vi "prerequisites_to_start_sleep_detection.vi"(4 "Input \nparameters":T3={"Frame rate (ms)"=2000, "Worm strain"="N2", "Time t"=0, "State"=enum."Image acquisition", "Acquisition time"=0, "Max_num_runs"=100000, "#TTL"=0, "SD start reference time"=100000, "ImSub Value"=0, "Time of last TTL"=0, "Number of Columns"=2, "Number of Rows"=2, "# AdjacentTTL"=0, "Start sleep detection"="", "Sleep Detection"=FALSE, "# Sleep detections"=0, "Time of first sleep detection"=0, "Time max # adjacent TTL"=0, "Image t-1"=[], "Image t"=[]} {"Number of Rows" items=["1"=1, "2"=2, "3"=3, "4"=4]; "Number of Columns" items=["1"=1, "2"=2, "3"=3, "4"=4]}, 6 "Deprivation\nparameters":T1={"Frame Row"=0, "Kstd"=40.0, "# Images for\nsleep detection"=10, "Kmean"=1.5, "Start time of sleep detection"=1000, 0, "Max deprivation length"=3600, "Max # TTL"=10000, "Delay detection start by x images after first detection"=0, "Minimum Interval between TTL pulses"=0, "Delay sleep detection\nby x detections"=9, "# Total immobility\n detections"=0.0, "Pause max # adjacent\nTTL"=0, "TTL x start\ntime deprivation\n"=0.0, "Max #\nadjacent TTL"=10000, " Ca2+\nmode"=0} {"?" items=["1", "2", "3", "4"]; "Frame Row" items=["1", "2", "3", "4"]}) -> (1 "Output \nparameters":T4={"Frame rate (ms)"=2000, "Worm strain"="N2", "Time t"=0, "State"=enum."Image acquisition", "Time elapsed"=0.0, "Max_num_runs"=100000, "#TTL"=0, "SD start reference"=100000, "ImSub Value"=0, "Time of last TTL"=0, "Number of Columns"=2, "Number of Rows"=2, "# AdjacentTTL"=0, "Start sleep detection"="", "Sleep Detection"=FALSE, "# Sleep detections"=0, "Time of first sleep detection"=0, "Time max # adjacent TTL"=0, "Image t-1"=[], "Image t"=[]} {"Number of Rows" items=["1"=1, "2"=2, "3"=3, "4"=4]; "Number of Columns" items=["1"=1, "2"=2, "3"=3, "4"=4]})   [LabVIEW 2011]
uses:
  state.ctl
panel:
  # "Sleep deprivation settings"
  # "Select deprivation animal"
  # "Deprive image in row"
  # "Deprive image in column"
  # "Sleep detection parameters"
  # "Sleep deprivation parameters"
  # "Delay deprivation start:"
  # "Pause deprivation (images):"
  # "Stop deprivation after:"
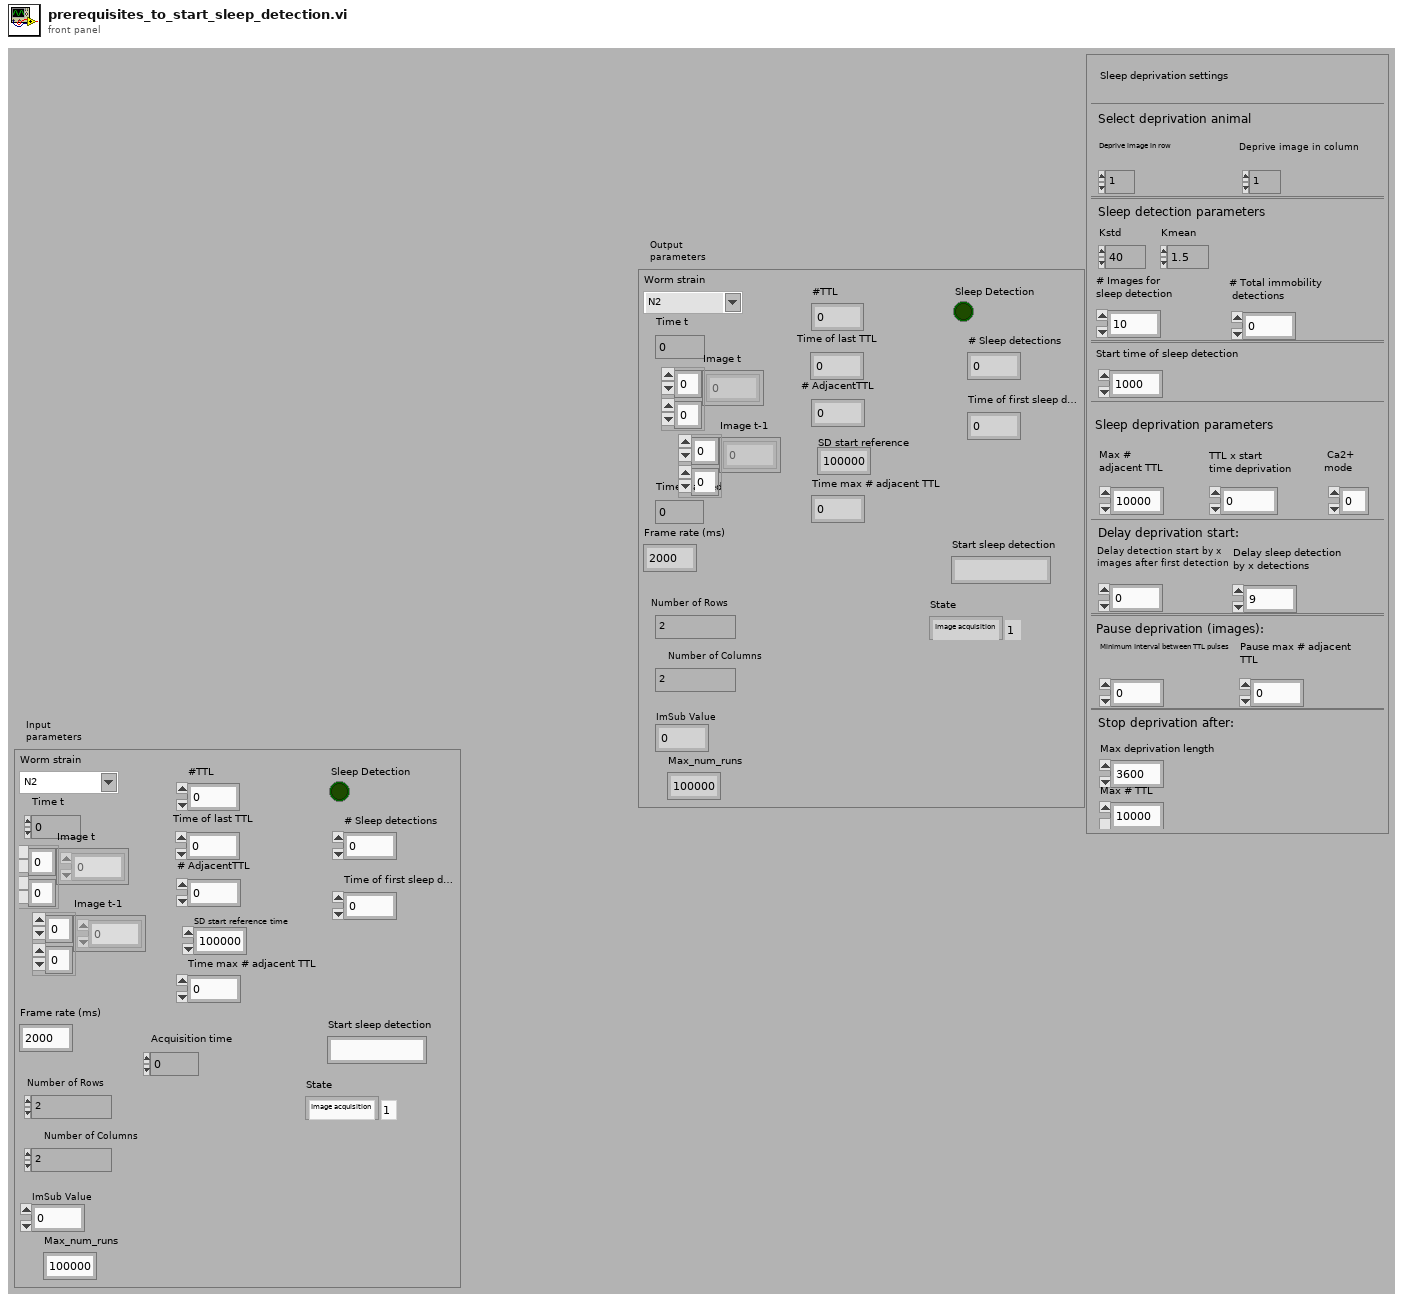
[diagram p1: front panel]
types:
  T1 = cluster{"Frame Row":u32, "Kstd":dbl, "# Images for\nsleep detection":i32, "Kmean":dbl, "Start time of sleep detection":i32, u32, "Max deprivation length":i32, "Max # TTL":i32, "Delay detection start by x images after first detection":i32, "Minimum Interval between TTL pulses":i32, "Delay sleep detection\nby x detections":i32, "# Total immobility\n detections":dbl, "Pause max # adjacent\nTTL":i32, "TTL x start\ntime deprivation\n":dbl, "Max #\nadjacent TTL":i32, " Ca2+\nmode":i32}
  T2 = typedef "state.ctl" = enum16{"Initialize measurement", "Image acquisition", "Image processing", "Sleep detection", "Control TTL protocol ", "Sleep deprivation", "Update image & exit condition", "Wait "}
  T3 = cluster{"Frame rate (ms)":u32, "Worm strain":string, "Time t":i32, "State":T2, "Acquisition time":i32, "Max_num_runs":i32, "#TTL":i32, "SD start reference time":i32, "ImSub Value":i32, "Time of last TTL":i32, "Number of Columns":u32, "Number of Rows":u32, "# AdjacentTTL":i32, "Start sleep detection":string, "Sleep Detection":bool, "# Sleep detections":i32, "Time of first sleep detection":i32, "Time max # adjacent TTL":i32, "Image t-1":i32[][], "Image t":i32[][]}
  T4 = cluster{"Frame rate (ms)":u32, "Worm strain":string, "Time t":i32, "State":T2, "Time elapsed":dbl, "Max_num_runs":i32, "#TTL":i32, "SD start reference":i32, "ImSub Value":i32, "Time of last TTL":i32, "Number of Columns":u32, "Number of Rows":u32, "# AdjacentTTL":i32, "Start sleep detection":string, "Sleep Detection":bool, "# Sleep detections":i32, "Time of first sleep detection":i32, "Time max # adjacent TTL":i32, "Image t-1":i32[][], "Image t":i32[][]}
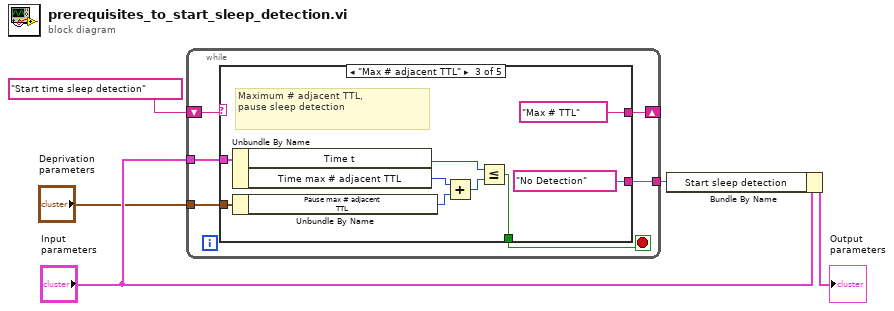
[diagram p0: block diagram]
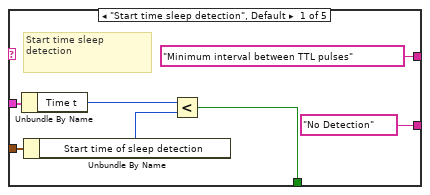
[diagram p2: hidden frame]
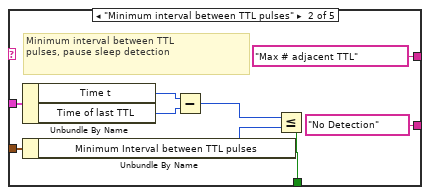
[diagram p3: hidden frame]
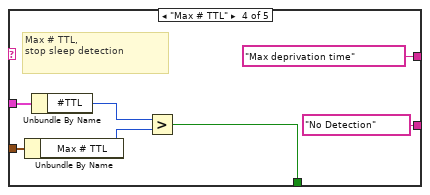
[diagram p4: hidden frame]
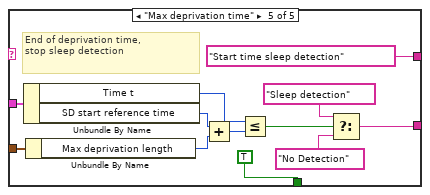
[diagram p5: hidden frame]
diagram:
  n1 = while {
    tunnel: "Deprivation\nparameters" -> [w11]
    tunnel: "Input \nparameters" -> [w10]
    shift-right: [w7] -> _
    shift-left: "Start time sleep detection" -> [w8]
    tunnel: [w6] -> w4
    stop <- w9 stop-if-true
    n2 = case shown="\"Max # adjacent TTL\"" w8 {
      tunnel: w11 -> [w18 w20 w31 w43 w55]
      tunnel: w10 -> [w17 w25 w36 w42 w54]
      tunnel: [w14 w21 w34 w37 TRUE] -> w9
      tunnel: ["Minimum interval between TTL pulses" "Max # adjacent TTL" "Max # TTL" "Max deprivation time" "Start time sleep detection"] -> w7
      tunnel: ["No Detection" "No Detection" "No Detection" "No Detection" w47] -> w6
      frame "Start time sleep detection", Default {
        # "Start time sleep detection"
        n3 = Unbundle By Name(w17) -> ("Time t"=w15:i32)
        n4 = Unbundle By Name(w18) -> ("Start time of sleep detection"=w16:i32)
        n5 = Less?(x=w15, y=w16) -> (x < y?=w14:bool)
      }
      frame "Minimum interval between TTL pulses" {
        # "Minimum interval between TTL\npulses, pause sleep detection"
        n6 = Unbundle By Name(w25) -> ("Time t"=w23:i32, "Time of last TTL"=w24:i32)
        n7 = Unbundle By Name(w20) -> ("Minimum Interval between TTL pulses"=w19:i32)
        n8 = Subtract(x=w23, y=w24) -> (x-y=w22:i32)
        n9 = Less Or Equal?(x=w22, y=w19) -> (x <= y?=w21:bool)
      }
      frame "Max # adjacent TTL" {
        # "Maximum # adjacent TTL,\npause sleep detection"
        n10 = Unbundle By Name(w36) -> ("Time t"=w35:i32, "Time max # adjacent TTL"=w30:i32)
        n11 = Unbundle By Name(w31) -> ("Pause max # adjacent\nTTL"=w29:i32)
        n12 = Add(x=w30, y=w29) -> (x+y=w28:i32)
        n13 = Less Or Equal?(x=w35, y=w28) -> (x <= y?=w34:bool)
      }
      frame "Max # TTL" {
        # "Max # TTL,\nstop sleep detection"
        n14 = Unbundle By Name(w43) -> ("Max # TTL"=w38:i32)
        n15 = Unbundle By Name(w42) -> ("#TTL"=w39:i32)
        n16 = Greater?(x=w39, y=w38) -> (0:w37:bool)
      }
      frame "Max deprivation time" {
        # "End of deprivation time,\nstop sleep detection"
        n17 = Unbundle By Name(w54) -> ("Time t"=w50:i32, "SD start reference time"=w52:i32)
        n18 = Unbundle By Name(w55) -> ("Max deprivation length"=w53:i32)
        n19 = Add(x=w52, y=w53) -> (x+y=w51:i32)
        n20 = Less Or Equal?(x=w50, y=w51) -> (x <= y?=w46:bool)
        n21 = Select(t="Sleep detection", s=w46, f="No Detection") -> (s? t:f=w47:string)
      }
    }
  }
  n22 = Bundle By Name(cluster="Input \nparameters", "Start sleep detection"=w4) -> (→"Output \nparameters":T3)
